vi "Module Timeout--constant.vi"() -> (3 "Module Timeout":i32)   [LabVIEW 2018, in "HW Interaction.lvlib"]
doc: "A module-wide common value to use as the timeout for various synchronization actions.\n_____\nBased on Delacor QMH Project Template 4.2.1.64."
uses:
  HW Interaction.lvlib
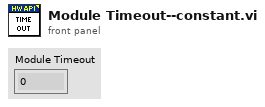
[diagram p1: front panel]
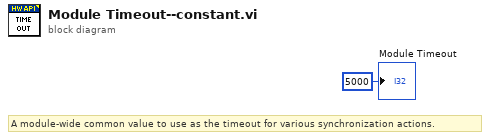
[diagram p0: block diagram]
diagram:
  # "A module-wide common value to use as the timeout for various synchronization actions."
  "Module Timeout" <- 5000 ("Module Timeout")
